vi "Initialize.vi"(8 "error in":errorcluster, 9 "Reset":i32(ring) items=["Reset Device", "Don't Reset"], 10 "ID Query":i32(ring) items=["Do Query", "Skip Query"], 11 "Resource Name":string) -> (0 "error out":errorcluster, 3 "Instr Handle":i32 caption="Instrument Handle")   [LabVIEW 8.6, in "ZTScopeM.lvlib"]
doc: "Establish an instrument communication session."
uses:
  ZTScopeM.lvlib
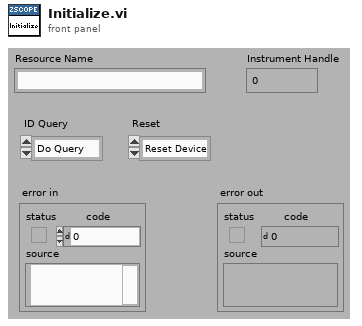
[diagram p1: front panel]
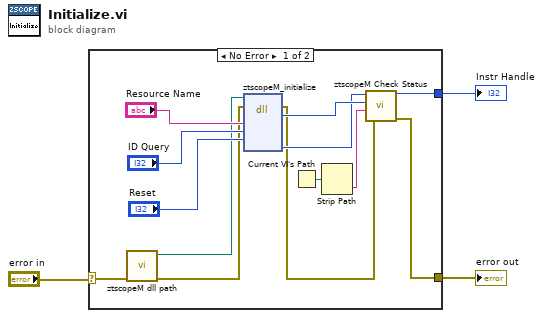
[diagram p0: block diagram]
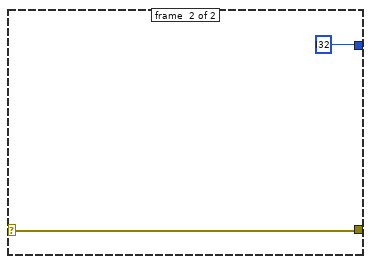
[diagram p2: hidden frame]
diagram:
  n1 = case shown="No Error" "error in" {
    selector: "error in" -> [w7 w17]
    tunnel: [w8 w17] -> w2
    tunnel: [w9 i32 ? ("instrumentHandle")] -> w1
    frame #0 {
      n2 = call "ztscopeM dll path.vi"("error in (no error)"=w7) -> ("error out"=w5:errorcluster, "<instrument>.dll path"=w6:path)  [unwired: 9 in]
      n3 = dll-call lib="C:/Program Files (x86)/National Instruments/LabVIEW 2013/instr.lib/ztscopem/ztscopeM.dll" fn="ztscopeM_initialize"(path in=w6, error in=w5, "resourceName"="Resource Name", "IDQuery"="ID Query", "reset"="Reset") -> (error out=w4:errorcluster, w13:i32, "instrumentHandle"=w12:i32)  [unwired: 5 in, 1 out]
      n4 = Current VI's Path() -> (path=w11:path)
      n5 = Strip Path(path=w11) -> (name=w10:string)  [unwired: 1 out]
      n6 = call "ztscopeM Check Status.vi"("error in"=w4, "name of VI"=w10, "status (return code)"=w13, "instrument handle in"=w12) -> ("error out"=w8:errorcluster, "instrument handle out"=w9:i32)  [unwired: 2 in]
    }
    frame #1 {
    }
  }
  "Instr Handle" <- w1
  "error out" <- w2
